vi "Prime BSI Open Close Library.vi"(0 "Open Library?":bool, 11 "Error In":errorcluster) -> (4 "Cameras Ref":refnum<k24>, 8 "Library Ref":refnum<k24>, 15 "Error Out":errorcluster)   [LabVIEW 2020]
uses:
  C:/Users/Public/Documents/Photometrics/TPM-LabVIEWSamples/Examples/2020/Dependencies/PVCamNET.dll
  Public/Documents/Photometrics/TPM-LabVIEWSamples/Examples/2020/Dependencies/PVCamNET.dll
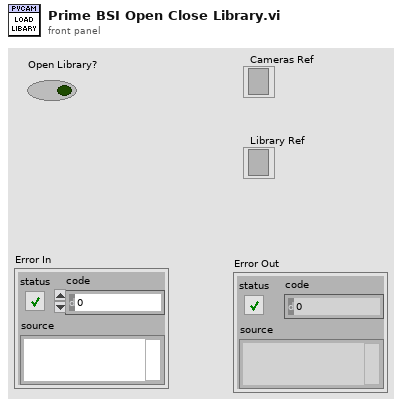
[diagram p1: front panel]
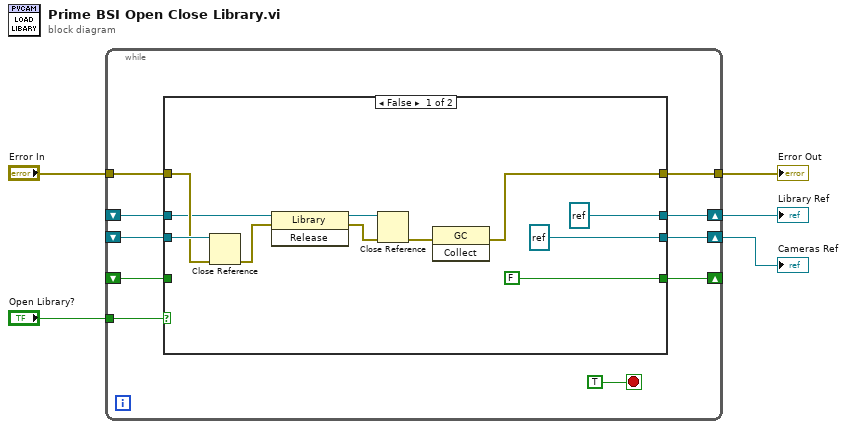
[diagram p0: block diagram]
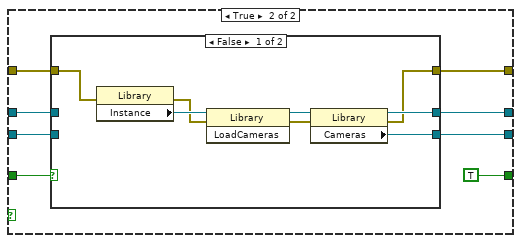
[diagram p2: hidden frame]
diagram:
  n1 = while {
    shift-right: [w13] -> w5
    shift-left: _ -> [w12]
    shift-right: [w14] -> w4
    shift-left: _ -> [w11]
    tunnel: "Error In" -> [w10]
    tunnel: [w9] -> w2
    tunnel: "Open Library?" -> [w8]
    shift-right: [w6] -> _
    shift-left: _ -> [w7]
    stop <- TRUE stop-if-true
    n2 = case shown="False" w8 {
      tunnel: [refnum<k24> refnum ("Instance") w34] -> w13
      tunnel: [refnum<k24> refnum ("Cameras") w33] -> w14
      tunnel: w12 -> [w20 w28]
      tunnel: w11 -> [w25 w27]
      tunnel: w10 -> [w24 w31]
      tunnel: [w18 w32] -> w9
      tunnel: w7 -> [_ w29]
      tunnel: [FALSE TRUE] -> w6
      frame False {
        n3 = Close Reference(reference=w25, error in (no error)=w24) -> (error out=w19:errorcluster)
        n4 = invoke class="Library" method="Release"(reference=w20, error in=w19) -> (reference out=w23:refnum<k24>, error out=w22:errorcluster)  [unwired: 1 in, 1 out]
        n5 = Close Reference(reference=w23, error in (no error)=w22) -> (error out=w21:errorcluster)
        n6 = invoke class="GC" method="Collect"(error in=w21) -> (error out=w18:errorcluster)  [unwired: 2 in, 2 out]
      }
      frame True {
        n7 = case shown="False" w29 {
          tunnel: [w41 w45] -> w34
          tunnel: [w40 w44] -> w33
          tunnel: [w39 w43] -> w32
          tunnel: w31 -> [w35 w43]
          tunnel: w28 -> [_ w45]
          tunnel: w27 -> [_ w44]
          frame False {
            n8 = property class="Library"(error in=w35) -> (error out=w36:errorcluster, "Instance"=w42:refnum<k24>)  [unwired: 1 in, 1 out]
            n9 = invoke class="Library" method="LoadCameras"(reference=w42, error in=w36) -> (reference out=w37:refnum<k24>, error out=w38:errorcluster)  [unwired: 1 in, 1 out]
            n10 = property class="Library"(reference=w37, error in=w38) -> (reference out=w41:refnum<k24>, error out=w39:errorcluster, "Cameras"=w40:refnum<k24>)
          }
          frame True {
          }
        }
      }
    }
  }
  "Library Ref" <- w5
  "Cameras Ref" <- w4
  "Error Out" <- w2
